vi "Publish Server Status.vi"(8 "error in (no error)":errorcluster, 11 "System Configuration":T1) -> (0 "error out":errorcluster, 3 "dup System Configuration":T1)   [LabVIEW 2024]
doc: "Publishes the server status with shared variables."
uses:
  Controls/Server/System Configuration.ctl
  Controls/Server/Subsystem Configuration.ctl
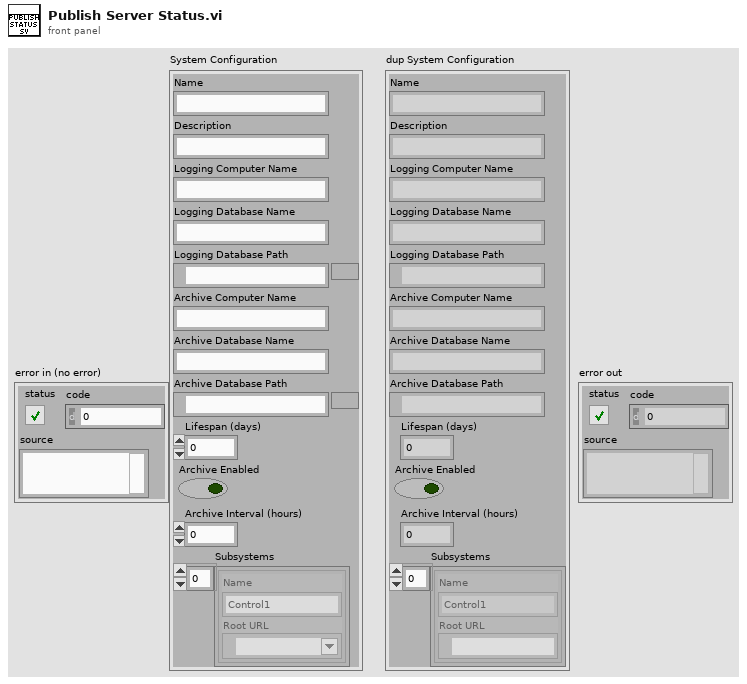
[diagram p1: front panel]
types:
  T1 = typedef "System Configuration.ctl" = cluster{"Name":string, "Description":string, "Logging Computer Name":string, "Logging Database Name":string, "Logging Database Path":path, "Archive Computer Name":string, "Archive Database Name":string, "Archive Database Path":path, "Lifespan (days)":u32, "Archive Enabled":bool, "Archive Interval (hours)":u32, "Subsystems":T2[]}
  T2 = typedef "Subsystem Configuration.ctl" = cluster{"Name":string, "Root URL":refnum<k21>}
  T3 = enum32{"u32BitField", "bool", "double", "string", "int8", "uint8", "int16", "uint16", "int32", "uint32", "int64", "uint64", "single", "double waveform", "int16 waveform", "array of boolean", "array of int8", "array of uint8", "array of int16", "array of uint16", "array of int32", "array of uint32", "array of int64", "array of uint64", "array of single", "array of double", "array of double waveform", "array of int16 waveform", "array of string", "variant", "timestamp", "fixed point", "custom"}
  T4 = cluster{"format string":string, "data type":enum32{"u32BitField", "bool", "double", "string", "int8", "uint8", "int16", "uint16", "int32", "uint32", "int64", "uint64", "single", "double waveform", "int16 waveform", "array of boolean", "array of int8", "array of uint8", "array of int16", "array of uint16", "array of int32", "array of uint32", "array of int64", "array of uint64", "array of single", "array of double", "array of double waveform", "array of int16 waveform", "array of string", "variant", "timestamp", "fixed point", "custom"}}
  T5 = cluster{"format string":string, "data type":enum32{"u32BitField", "bool", "double", "string", "int8", "uint8", "int16", "uint16", "int32", "uint32", "int64", "uint64", "single", "double waveform", "int16 waveform", "array of boolean", "array of int8", "array of uint8", "array of int16", "array of uint16", "array of int32", "array of uint32", "array of int64", "array of uint64", "array of single", "array of double", "array of double waveform", "array of int16 waveform", "array of string", "variant", "timestamp", "fixed point", "custom"}}[]
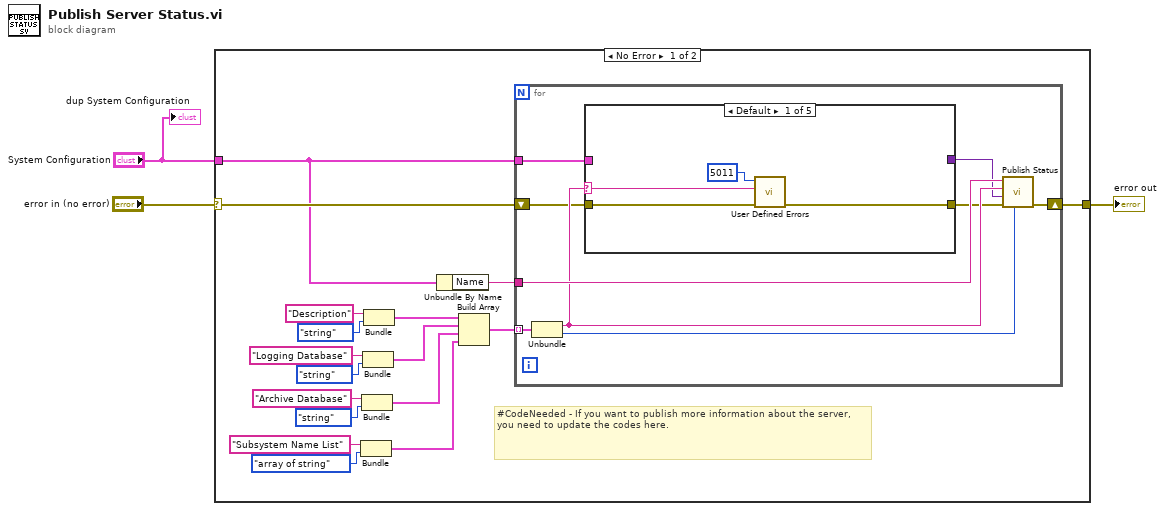
[diagram p0: block diagram]
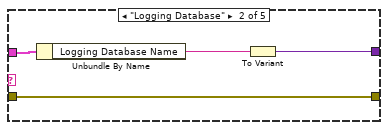
[diagram p2: hidden frame]
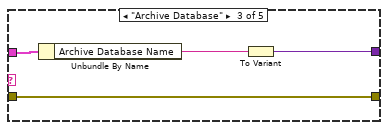
[diagram p3: hidden frame]
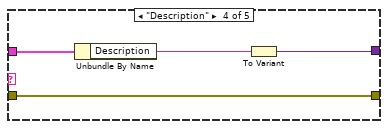
[diagram p4: hidden frame]
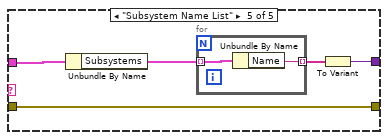
[diagram p5: hidden frame]
diagram:
  n1 = case shown="No Error" "error in (no error)" {
    selector: "error in (no error)" -> [w20 w53]
    tunnel: [w6 w53] -> w3
    tunnel: "System Configuration" -> [w5 _]
    frame No Error {
      # "#CodeNeeded - If you want to publish more information about the server, you need to update the codes here."
      n2 = Bundle("format string"="Subsystem Name List", "data type"=T3."array of string") -> (w7:T4)  [unwired: 1 in]
      n3 = Bundle("format string"="Archive Database", "data type"=T3."string") -> (w10:T4)  [unwired: 1 in]
      n4 = Bundle("format string"="Logging Database", "data type"=T3."string") -> (w13:T4)  [unwired: 1 in]
      n5 = Bundle("format string"="Description", "data type"=T3."string") -> (w16:T4)  [unwired: 1 in]
      n6 = Unbundle By Name(w5) -> ("Name"=w4:string)
      n7 = Build Array(w16, w13, w10, w7) -> (w19:T5)
      n8 = for {
        tunnel: w19 -> [w29] mode=indexing
        shift-right: [w27] -> w6
        shift-left: w20 -> [w22]
        tunnel: w5 -> [w28]
        tunnel: w4 -> [w26]
        n9 = Unbundle(w29) -> ("format string"=w24:string, "data type"=w25:T3)
        n10 = case shown="Default" w24 {
          selector: w24 -> [w31 _ _ _ _]
          tunnel: w28 -> [_ w36 w40 w44 w50]
          tunnel: [_ w34 w38 w42 w47] -> w23
          tunnel: w22 -> [w33 w37 w41 w45 w46]
          tunnel: [w32 w37 w41 w45 w46] -> w21
          frame Default {
            n11 = call "User Defined Errors.vi"("error in (no error)"=w33, "Parameter 1"=w31, "Error Code (0)"=5011 ("error code (0)")) -> ("error out"=w32:errorcluster)  [unwired: 8 in]
          }
          frame "Logging Database" {
            n12 = Unbundle By Name(w36) -> ("Logging Database Name"=w35:string)
            n13 = To Variant(anything=w35) -> (Variant=w34:variant)
          }
          frame "Archive Database" {
            n14 = Unbundle By Name(w40) -> ("Archive Database Name"=w39:string)
            n15 = To Variant(anything=w39) -> (Variant=w38:variant)
          }
          frame "Description" {
            n16 = Unbundle By Name(w44) -> ("Description"=w43:string)
            n17 = To Variant(anything=w43) -> (Variant=w42:variant)
          }
          frame "Subsystem Name List" {
            n18 = Unbundle By Name(w50) -> ("Subsystems"=w49:T2[])
            n19 = for {
              tunnel: [w52] -> w48 mode=indexing
              tunnel: w49 -> [w51] mode=indexing
              n20 = Unbundle By Name(w51) -> ("Name"=w52:string)
            }
            n21 = To Variant(anything=w48) -> (Variant=w47:variant)
          }
        }
        n22 = call "Publish Status.vi"("Data Type"=w25, "error in (no error)"=w21, "Value"=w23, "Parameter"=w24, "System Name"=w26) -> ("error out"=w27:errorcluster)  [unwired: 6 in]
      }
    }
    frame Error {
    }
  }
  "error out" <- w3
  "dup System Configuration" <- "System Configuration"
